vi "Initialize.vi"(8 "error in (no error)":errorcluster, 10 "dynamic parameters":T2[](array[typedef]), 11 "SR6-NC Arm":T1={"L1x"=0.19, "L1y"=0.51, "L2"=0.6, "L3"=0.105, "L4"=0.6, "L6"=0.085}) -> (0 "error out":errorcluster, 3 "SR6-NC Arm out":refnum<class "SR6-NC Arm.lvclass">)   [LabVIEW 2013, in "SR6-NC Arm.lvclass"]
uses:
  SR6-NC Arm.lvclass
  <vilib>/robotics/Kinematics/DH Dynamic Parameters.ctl
  <vilib>/Analysis/Matrix/Datatypes/RealMatrix.ctl
  <vilib>/robotics/Kinematics/DH Kinematic Parameters.ctl
  <vilib>/robotics/Kinematics/Link/Joint Type.ctl
  <vilib>/robotics/Kinematics/Link/NI_Robotics_Link.lvclass
  <vilib>/Analysis/_algsub.llb/Vector Norm.vi
  <vilib>/Analysis/_algsub.llb/Real Vector Norm.vi
  <vilib>/Analysis/baseanly.llb/Outer Product.vi
  <vilib>/Analysis/baseanly.llb/Real Outer Product.vi
  <vilib>/robotics/Kinematics/Create Lie Group Matrix.vi
  <vilib>/Analysis/7linalg.llb/Create Special Matrix.vi
  <vilib>/Analysis/7linalg.llb/Create Special Real Matrix.vi
  <vilib>/Analysis/Matrix/Numeric/Multiply/Multiply.vi
  <vilib>/Analysis/Matrix/Numeric/Multiply/Multiply - RM,R.vi
  <vilib>/Analysis/Matrix/Numeric/Multiply/Multiply - R,RM.vi
  <vilib>/Analysis/Matrix/Numeric/Add/Add.vi
  <vilib>/Analysis/Matrix/Numeric/Add/Add - RM,RM.vi
  <vilib>/robotics/Kinematics/Robot/NI_Robotics_Serial Robot Arm.lvclass
  <vilib>/robotics/Utilities/NI_Robotics Utilities.lvlib
  <vilib>/robotics/Kinematics/NI_Kinematics.lvlib
  <vilib>/Analysis/Matrix/NI_Matrix.lvlib
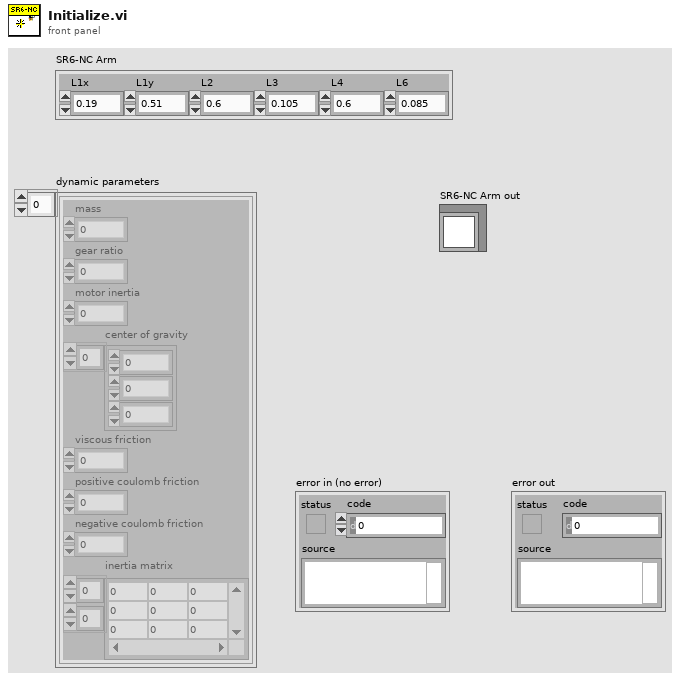
[diagram p1: front panel]
types:
  T1 = cluster{"L1x":dbl, "L1y":dbl, "L2":dbl, "L3":dbl, "L4":dbl, "L6":dbl}
  T2 = typedef "DH Dynamic Parameters.ctl" = cluster{"mass":dbl, "gear ratio":dbl, "motor inertia":dbl, "center of gravity":dbl[], "viscous friction":dbl, "positive coulomb friction":dbl, "negative coulomb friction":dbl, "inertia matrix":T3}
  T3 = typedef "NI_Matrix.lvlib/RealMatrix.ctl" = dbl[][]
  T4 = typedef "DH Kinematic Parameters.ctl" = cluster{"twist angle":dbl, "length":dbl, "rotation angle":dbl, "offset distance":dbl, "joint type":T5, "joint coordinate offset":dbl}
  T5 = typedef "NI_Robotics_Link.lvclass/Joint Type.ctl" = enum16{"Revolute", "Prismatic"}
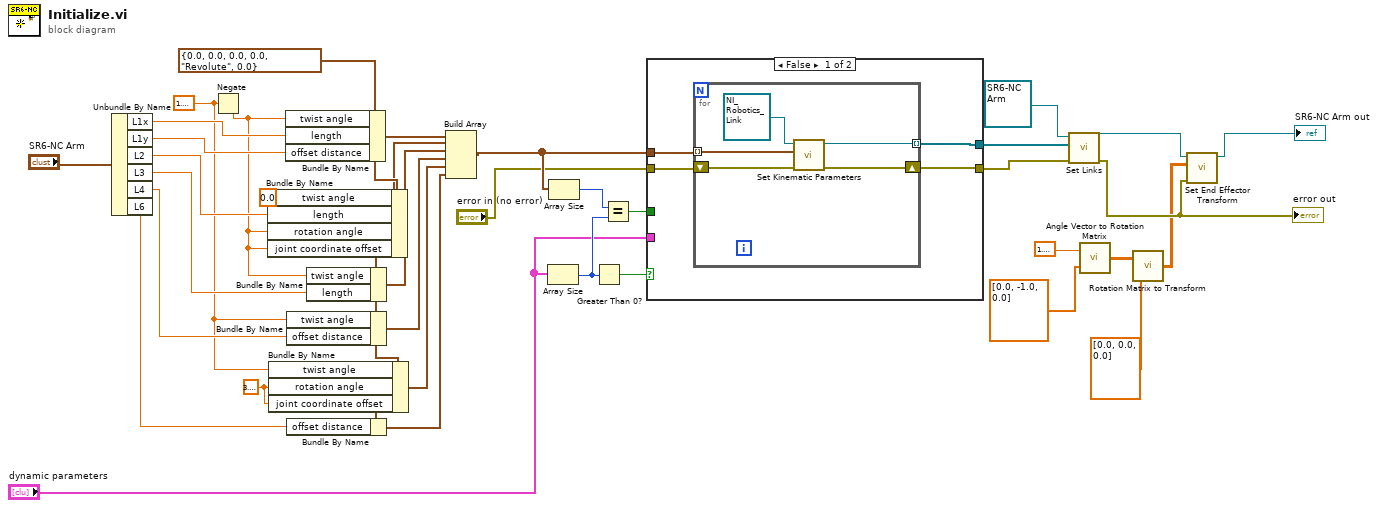
[diagram p0: block diagram]
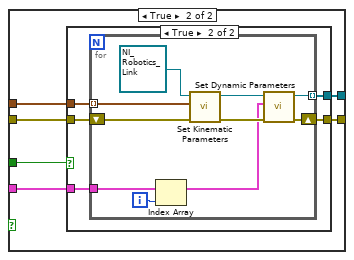
[diagram p2: hidden frame]
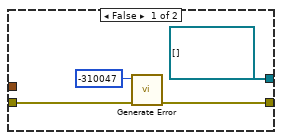
[diagram p3: hidden frame]
diagram:
  w9 = 3.141592653589793
  w10 = 1.5707963267948966
  w29 = T4 {"twist angle"=0.0, "length"=0.0, "rotation angle"=0.0, "offset distance"=0.0, "joint type"=enum."Revolute", "joint coordinate offset"=0.0} ("Link Parameters")
  n1 = Unbundle By Name("SR6-NC Arm") -> ("L1x"=w35:dbl, "L1y"=w34:dbl, "L2"=w32:dbl, "L3"=w31:dbl, "L4"=w30:dbl, "L6"=w28:dbl)
  n2 = Negate(x=w10) -> (-x=w11:dbl)
  n3 = Bundle By Name(cluster=w29, "twist angle"=0.0, "length"=w32, "rotation angle"=w11, "joint coordinate offset"=w11) -> (w26:T4)
  n4 = Bundle By Name(cluster=w29, "twist angle"=w10, "rotation angle"=w9, "joint coordinate offset"=w9) -> (w23:T4)
  n5 = Bundle By Name(cluster=w29, "twist angle"=w11, "length"=w35, "offset distance"=w34) -> (w27:T4)
  n6 = Bundle By Name(cluster=w29, "twist angle"=w10, "offset distance"=w30) -> (w24:T4)
  n7 = Bundle By Name(cluster=w29, "offset distance"=w28) -> (w22:T4)
  n8 = Bundle By Name(cluster=w29, "twist angle"=w11, "length"=w31) -> (w25:T4)
  n9 = Build Array(w27, w26, w25, w24, w23, w22) -> (w15:T4[])
  n10 = Array Size(array="dynamic parameters") -> (size(s)=w17:i32)
  n11 = Array Size(array=w15) -> (size(s)=w18:i32)
  n12 = Greater Than 0?(x=w17) -> (x > 0?=w19:bool)
  n13 = Equal?(x=w18, y=w17) -> (x = y?=w16:bool)
  n14 = case shown="False" w19 {
    tunnel: w15 -> [w40 w51]
    tunnel: "error in (no error)" -> [w39 w50]
    tunnel: [w37 w49] -> w21
    tunnel: [w38 w48] -> w20
    tunnel: "dynamic parameters" -> [_ w47]
    tunnel: w16 -> [_ w46]
    frame False {
      n15 = for {
        tunnel: w40 -> [w44] mode=indexing
        shift-right: [w41] -> w37
        shift-left: w39 -> [w43]
        tunnel: [w42] -> w38 mode=indexing
        n16 = call <vilib>:"Set Kinematic Parameters.vi"("error in (no error)"=w43, "kinematic parameters"=w44, "link in"=refnum<class "NI_Robotics_Link.lvclass"> refnum ("Link")) -> ("error out"=w41:errorcluster, "link out"=w42:refnum<class "NI_Robotics_Link.lvclass">)  [unwired: 7 in]
      }
    }
    frame True {
      n17 = case shown="True" w46 {
        tunnel: w51 -> [_ w60]
        tunnel: w50 -> [w53 w59]
        tunnel: [w54 w58] -> w49
        tunnel: [refnum<class "NI_Robotics_Link.lvclass">[] [] w57] -> w48
        tunnel: w47 -> [_ w56]
        frame False {
          n18 = call <vilib>:"Generate Error.vi"("error in (no error)"=w53, "code"=-310047) -> ("error out"=w54:errorcluster)  [unwired: 9 in]
        }
        frame True {
          n19 = for {
            tunnel: w60 -> [w69] mode=indexing
            tunnel: w56 -> [w66]
            tunnel: [w64] -> w57 mode=indexing
            shift-right: [w65] -> w58
            shift-left: w59 -> [w63]
            i -> [w61]
            n20 = Index Array(array=w66, index=w61) -> (element=w62:T2)
            n21 = call <vilib>:"Set Kinematic Parameters.vi"("error in (no error)"=w63, "kinematic parameters"=w69, "link in"=refnum<class "NI_Robotics_Link.lvclass"> refnum ("Link")) -> ("error out"=w67:errorcluster, "link out"=w68:refnum<class "NI_Robotics_Link.lvclass">)  [unwired: 7 in]
            n22 = call <vilib>:"Set Dynamic Parameters.vi"("error in (no error)"=w67, "dynamic parameters"=w62, "link in"=w68) -> ("error out"=w65:errorcluster, "link out"=w64:refnum<class "NI_Robotics_Link.lvclass">)  [unwired: 7 in]
          }
        }
      }
    }
  }
  n23 = call <vilib>:"Set Links.vi"("error in (no error)"=w21, "links"=w20, "serial arm in"=refnum<class "SR6-NC Arm.lvclass"> refnum ("SR6-NC Arm out")) -> ("error out"=w5:errorcluster, "serial arm out"=w8:refnum<class "SR6-NC Arm.lvclass">)  [unwired: 7 out]
  "error out" <- w5
  n24 = call <vilib>:"Angle Vector to Rotation Matrix.vi"("vector"=dbl[] [0.0, -1.0, 0.0], "angle"=1.5707963267948966) -> ("rotation matrix"=w3:T3)
  n25 = call <vilib>:"Rotation Matrix to Transform.vi"("translation vector"=dbl[] [0.0, 0.0, 0.0], "rotation matrix"=w3) -> ("transform"=w1:T3)
  n26 = call <vilib>:"Set End Effector Transform.vi"("error in (no error)"=w5, "end effector transform"=w1, "serial arm in"=w8) -> ("serial arm out"=→"SR6-NC Arm out":refnum<class "SR6-NC Arm.lvclass">)  [unwired: 7 in, 1 out]
